vi "S7_StartCom.vi"(9 "ipAddress":string, 11 "siemens":i32(ring)=1 items=["S1200"=1, "S300"=2, "S400"=3, "S1500"=4, "S200Smart"=5, "S200"=6]) -> (0 "错误输出":errorcluster, 1 "IsSuccess":bool, 3 "connect id":refnum<k24>)   [LabVIEW 2018]
uses:
  E:/Fergus/S7/S7_code/Lib/HslCommunication.dll
  Lib/HslCommunication.dll
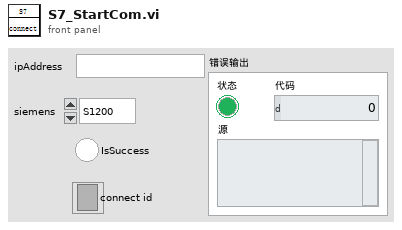
[diagram p1: front panel]
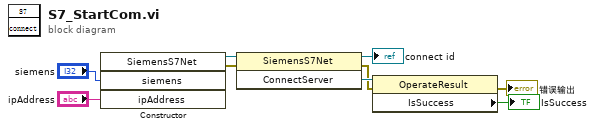
[diagram p0: block diagram]
diagram:
  n1 = constructor class="SiemensS7Net"("siemens"="siemens", "ipAddress"="ipAddress") -> (reference out=w9:refnum<k24>, error out=w3:errorcluster)  [unwired: 3 in, 3 out]
  n2 = invoke on="调用节点" class="SiemensS7Net" method="ConnectServer"(reference=w9, error in=w3) -> (reference out=→"connect id":refnum<k24>, error out=w2:errorcluster, "ConnectServer"=w8:refnum<k24>)  [unwired: 1 in]
  n3 = property on="属性节点" class="OperateResult"(reference=w8, error in=w2) -> (error out=→"错误输出":errorcluster, "IsSuccess"=→"IsSuccess":bool)  [unwired: 1 out]
